vi "Create Object (name).vi"(8 "error in (no error)":errorcluster, 11 "Name":string) -> (0 "error out":errorcluster, 3 "Scene:New Object":refnum<vi>)   [LabVIEW 2020, in "NI_3D Picture Control.lvlib"]
doc: "Creates a new 3D object to display in the 3D scene."
uses:
  NI_3D Picture Control.lvlib
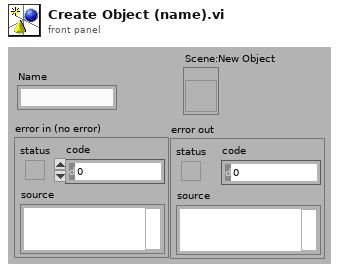
[diagram p1: front panel]
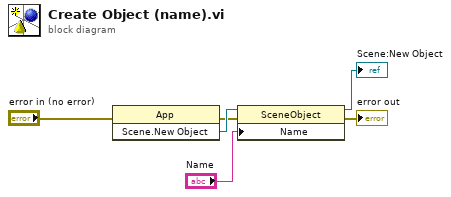
[diagram p0: block diagram]
diagram:
  n1 = invoke class="App" method="Scene.New Object"(error in="error in (no error)") -> (error out=w3:errorcluster, "Scene.New Object"=w5:refnum<vi>)  [unwired: 2 in, 1 out]
  n2 = property class="SceneObject"(reference=w5, error in=w3, "Name"="Name") -> (reference out=→"Scene:New Object":refnum<vi>, error out=→"error out":errorcluster)
